vi "Console_Facade.vi"(0 "Data In":T4, 2 "Display State In":T2, 3 "Container State":T3) -> (6 "Data Out":T4, 7 "Display State Out":T2, 8 "Action":T1)   [LabVIEW 2020, in "Console_Xctrl.xctl"]
uses:
  Console_Xctrl.xctl
  Console_Data.ctl
  <vilib>/_xctls/Container State.ctl
  Console_State.ctl
  <vilib>/_xctls/Action.ctl
  <vilib>/_xctls/XControlSupport.lvlib
panel:
  in  "String":string
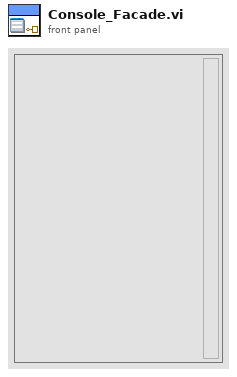
[diagram p1: front panel]
types:
  T1 = typedef "XControlSupport.lvlib/Action.ctl" = cluster{"Data Changed?":bool, "State Changed?":bool, "Action Name":string}
  T2 = typedef "Console_Xctrl.xctl/Console_State.ctl" = cluster{"Numeric":dbl}
  T3 = typedef "XControlSupport.lvlib/Container State.ctl" = cluster{"Indicator?":bool, "Run Mode?":bool, " Refnum":refnum<vi>}
  T4 = typedef "Console_Xctrl.xctl/Console_Data.ctl" = string
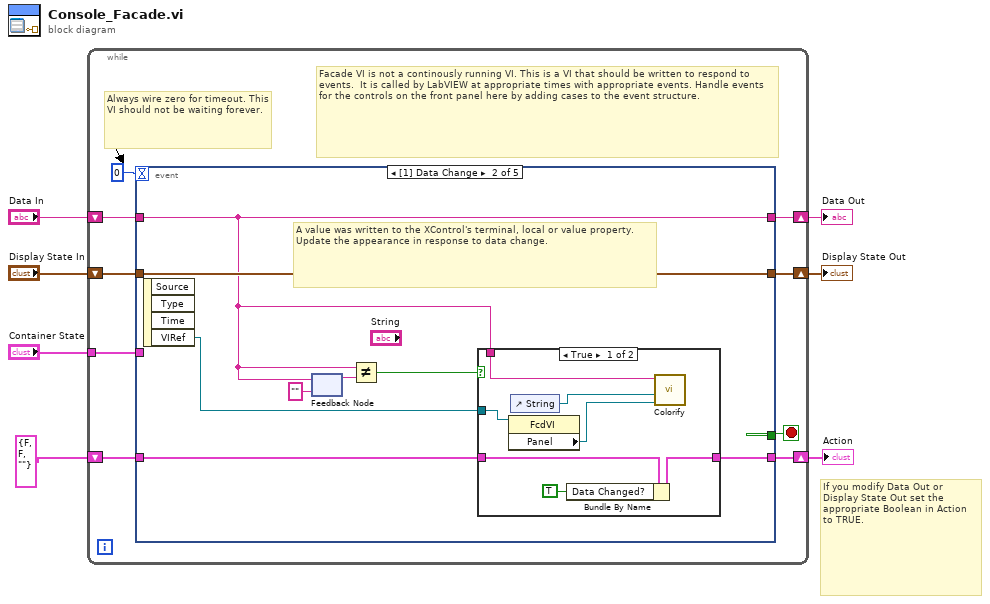
[diagram p0: block diagram]
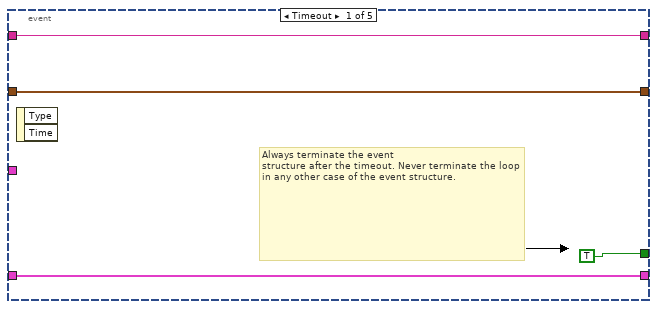
[diagram p2: hidden frame]
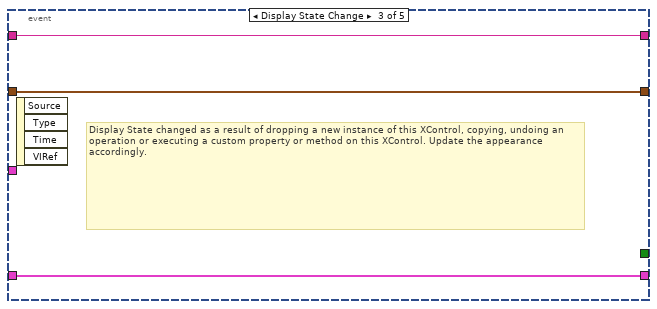
[diagram p4: hidden frame]
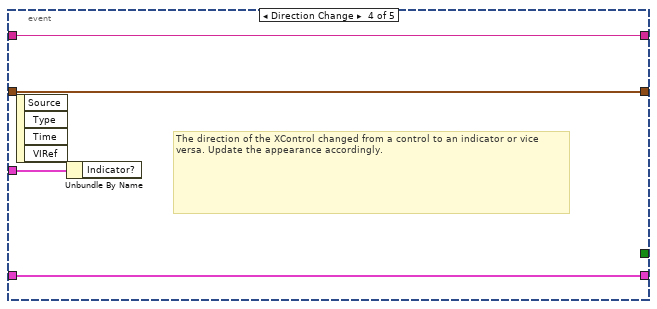
[diagram p5: hidden frame]
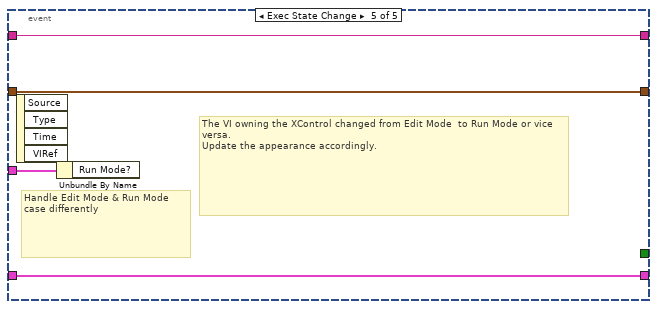
[diagram p6: hidden frame]
diagram:
  # "If you modify Data Out or\nDisplay State Out set the\nappropriate Boolean in Action\nto TRUE."
  n1 = while {
    shift-right: [w15] -> w4
    shift-left: "Display State In" -> [w16]
    tunnel: "Container State" -> [w12]
    shift-right: [w10] -> w7
    shift-left: "Data In" -> [w11]
    shift-right: [w8] -> w2
    shift-left: T1 {"Data Changed?"=FALSE, "State Changed?"=FALSE, "Action Name"=""} ("Action") -> [w9]
    stop <- w14 stop-if-true
    # "Facade VI is not a continously running VI. This is a VI that should be written to respond to events.  It is called by LabVIEW at appropriate times with appropriate events. Handle events for the controls on the front panel here by adding cases to the event structure."
    # "Always wire zero for timeout. This\nVI should not be waiting forever."
    n2 = event shown="[1] Data Change" {
      selector: _ -> [_ _ _ _ _]
      dyn-events: _ -> [_ _ _ _ _]
      timeout: 0 -> [_ _ _ _ _]
      tunnel: w16 -> [w18 w28 w39 w42 w46]
      tunnel: [w18 w28 w39 w42 w46] -> w15
      tunnel: [TRUE _ _ _ _] -> w14
      tunnel: w12 -> [_ _ _ w43 w47]
      tunnel: w11 -> [w17 w22 w38 w41 w45]
      tunnel: [w17 w22 w38 w41 w45] -> w10
      tunnel: [w19 w26 w37 w40 w44] -> w8
      tunnel: w9 -> [w19 w27 w37 w40 w44]
      event Timeout {
        # "Always terminate the event\nstructure after the timeout. Never terminate the loop in any other case of the event structure."
        n3 = event-data() -> ()  [unwired: 1 in, 2 out]
      }
      event Data Change {
        # "A value was written to the XControl's terminal, local or value property.\nUpdate the appearance in response to data change."
        n4 = event-data() -> ("VIRef"=w25:refnum<vi>)  [unwired: 1 in, 3 out]
        n5 = feedback-in #1(w22) -> ()
        n6 = feedback #1(T4 "" ("Data In")) -> (w23:T4)
        n7 = Not Equal?(x=w22, y=w23) -> (x != y?=w21:bool)
        n8 = case shown="True" w21 {
          tunnel: w27 -> [w35 w36]
          tunnel: [w33 w36] -> w26
          tunnel: w22 -> [w32 _]
          tunnel: w25 -> [w30 _]
          frame True {
            n9 = property class="FcdVI"(reference=w30) -> ("Panel"=w29:refnum<vi>)  [unwired: 1 in, 2 out]
            n10 = control-ref of="String"() -> (w31:refnum<vi>)
            n11 = Bundle By Name(cluster=w35, "Data Changed?"=TRUE) -> (w33:T1)
            n12 = call "Colorify.vi"("Front Panel"=w29, "String 2"=w31, "String"=w32) -> ()  [unwired: 9 in]
          }
          frame False {
          }
        }
      }
      event Display State Change {
        # "Display State changed as a result of dropping a new instance of this XControl, copying, undoing an operation or executing a custom property or method on this XControl. Update the appearance accordingly."
        n13 = event-data() -> ()  [unwired: 1 in, 4 out]
      }
      event Direction Change {
        # "The direction of the XControl changed from a control to an indicator or vice versa. Update the appearance accordingly."
        n14 = event-data() -> ()  [unwired: 1 in, 4 out]
        n15 = Unbundle By Name(w43) -> ()  [unwired: 1 out]
      }
      event Exec State Change {
        # "The VI owning the XControl changed from Edit Mode  to Run Mode or vice versa.\nUpdate the appearance accordingly."
        # "Handle Edit Mode & Run Mode\ncase differently"
        n16 = event-data() -> ()  [unwired: 1 in, 4 out]
        n17 = Unbundle By Name(w47) -> ()  [unwired: 1 out]
      }
    }
  }
  "Display State Out" <- w4
  "Data Out" <- w7
  "Action" <- w2
